vi "4Pi 4Pi Modes Control.vi"(7 "Calling VI Ref":refnum<vi>) -> ()   [LabVIEW 2016]
uses:
  4Pi 4Pi Modes - Controls/4Pi 4Pi Modes - Mirror Modes.ctl
  4Pi 4Pi Modes - Controls/4Pi 4Pi Modes - Standard Action.ctl
  <vilib>/Utility/miscctls.llb/LVPointTypeDef.ctl
  Hardware Configuration/Hardware Configuration Controls/Standard Action.ctl
  <vilib>/Analysis/baseanly.llb/Mean (DBL).vi
  <vilib>/Analysis/NI_AALBase.lvlib
  <userlib>/BMC/BMC.lvlib
panel:
  in  "Clear Flat":bool
  in  "Select Modes":bool
  in  "No Hardware":bool
  in  "Add Flat":bool
  out "?":string="Idel"
  out "?":string="Idel"
  in  "Set Astig":bool
  in  "Save Astig":bool
  out "Pixel Map (-1 to 1) 2":dbl[][](graph)
  in  "Scan Modes":bool
  in  "Astig On/Off":bool
  in  "Load Astig":bool
  in  "Clear Modes":bool
  in  "Mirror Modes":T1
  in  "Load Flat":bool
  in  "Save Flat":bool
  in  "Apply Flat":bool
  in  "Quit":bool
  out "Pixel Map (-1 to 1)":dbl[][](graph)
  # "Mode"
  # "Amount (nm)"
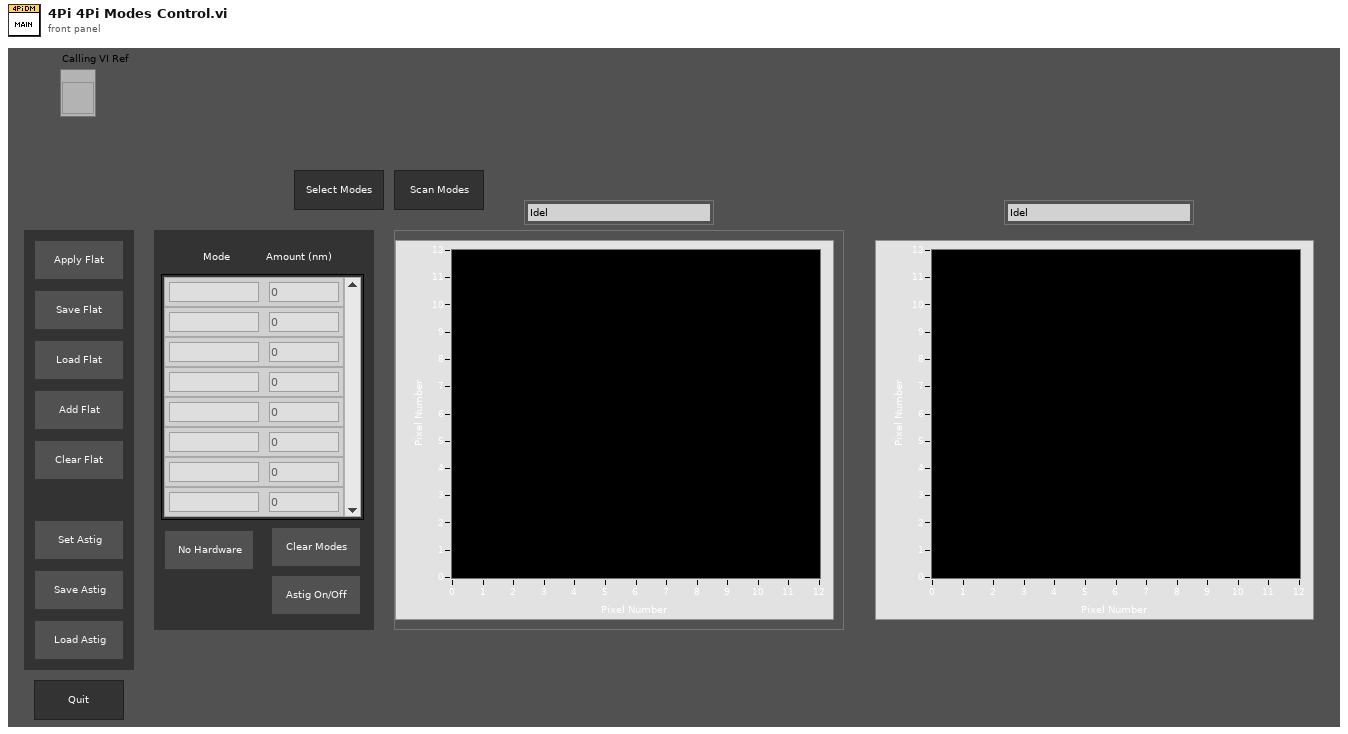
[diagram p1: front panel]
types:
  T1 = typedef "4Pi 4Pi Modes - Mirror Modes.ctl" = cluster{"Mode":string, "Amplitude":dbl}[]
  T2 = enum16{"Always On", "Always Off", "Off While Running"}
  T3 = typedef "LVPointTypeDef.ctl" = cluster{"Horizontal":i16, "Vertical":i16}
  T4 = typedef "4Pi 4Pi Modes - Standard Action.ctl" = enum16{"Read", "Write"}
  T5 = cluster{"type":i16, "ID":i16, "size":i32, "lutName":u64, "priv":u64}[]
  T6 = typedef "Standard Action.ctl" = enum16{"Read", "Write"}
  T7 = typedef "LVRectTypeDef.ctl" = cluster{"Left":i16, "Top":i16, "Right":i16, "Bottom":i16}
  T8 = typedef "LVBoundsTypeDef.ctl" = cluster{"Width":u32, "Height":u32}
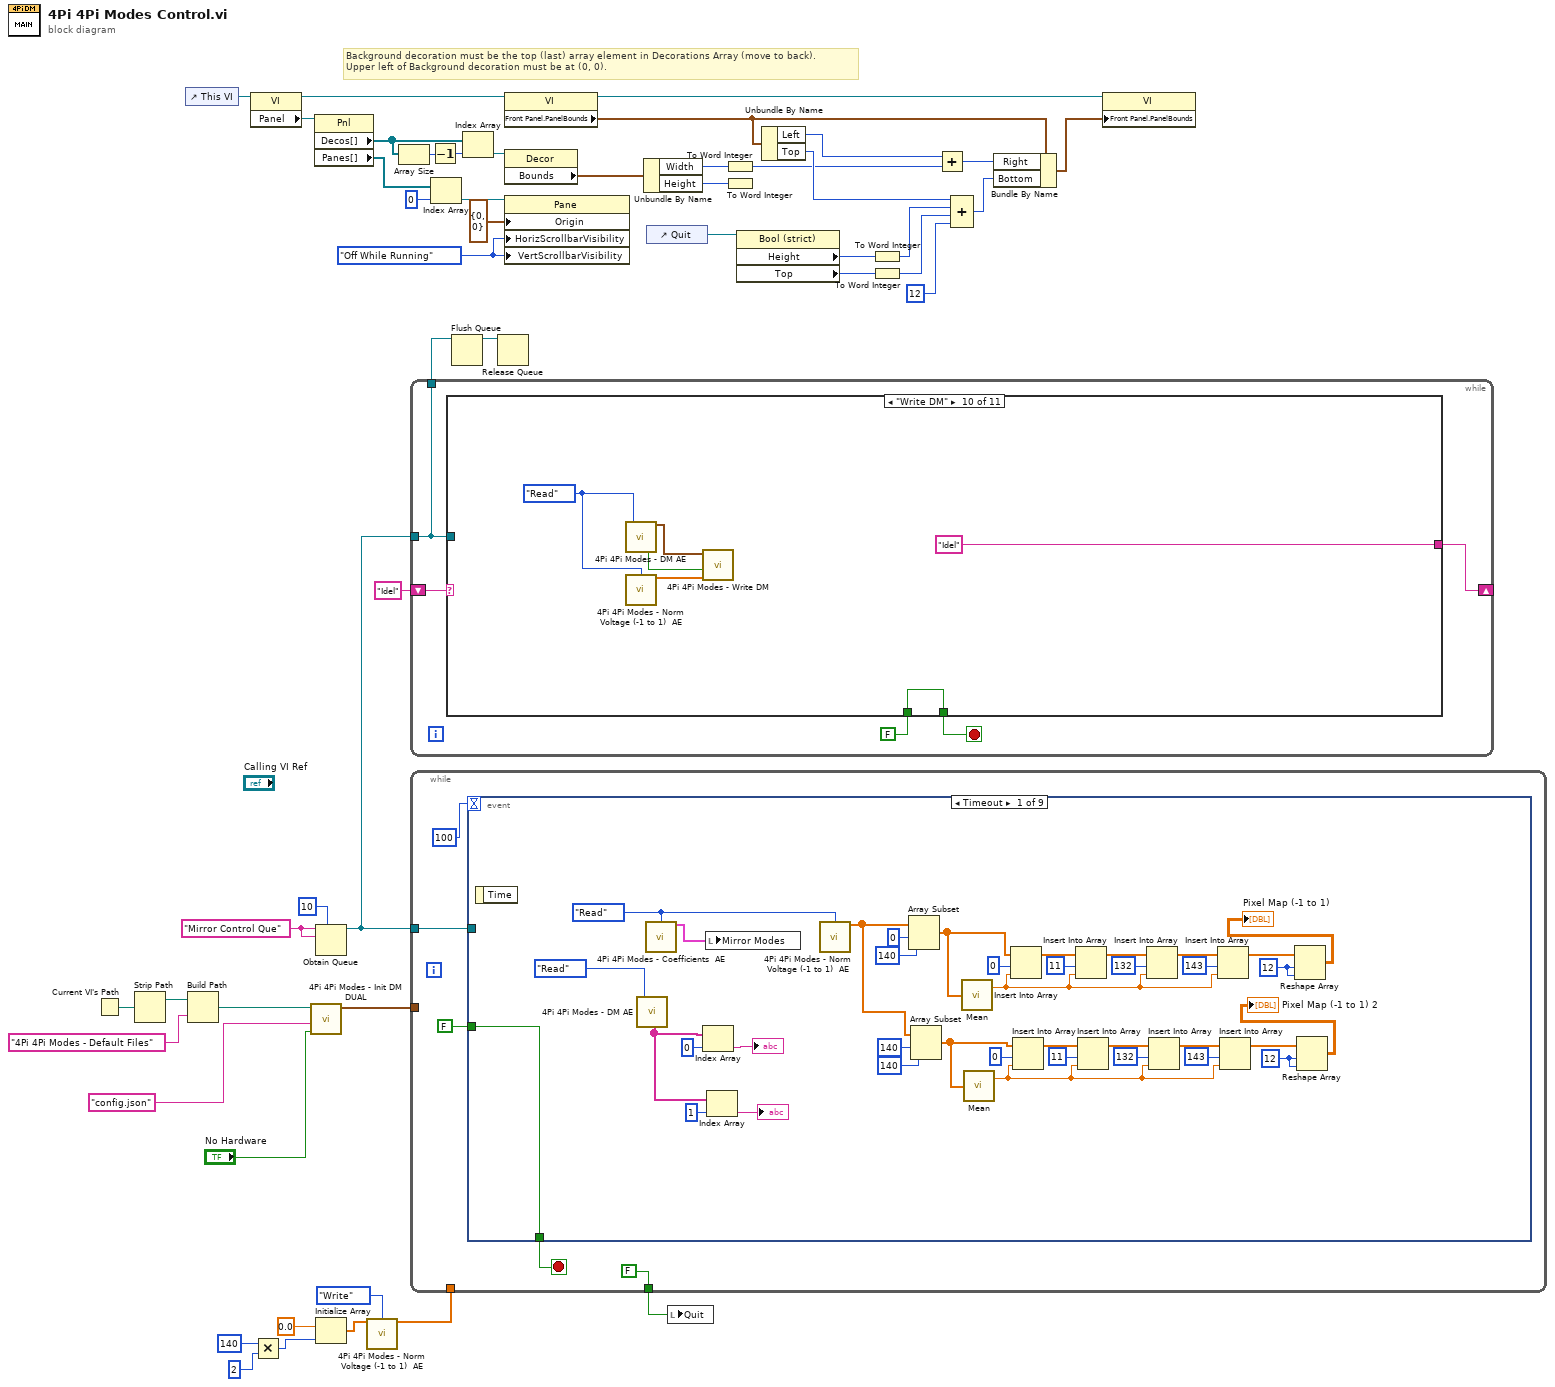
[diagram p0: block diagram]
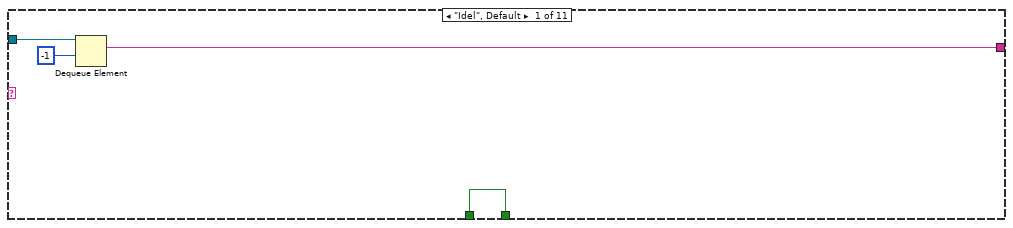
[diagram p2: hidden frame]
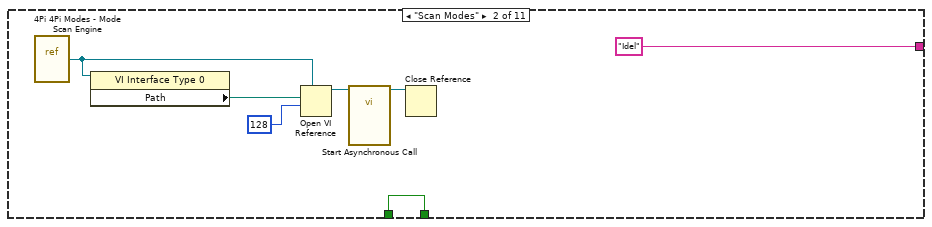
[diagram p3: hidden frame]
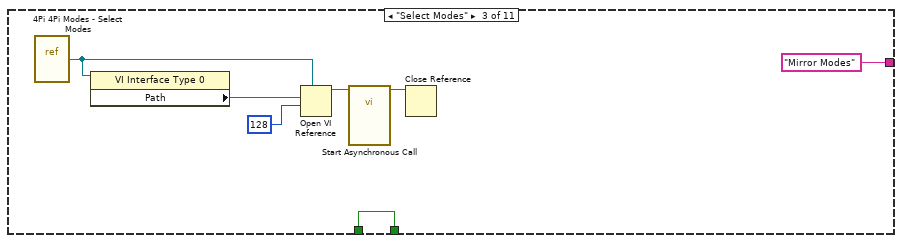
[diagram p4: hidden frame]
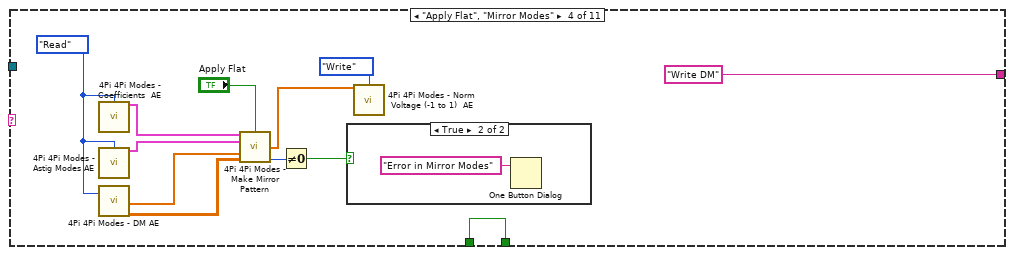
[diagram p5: hidden frame]
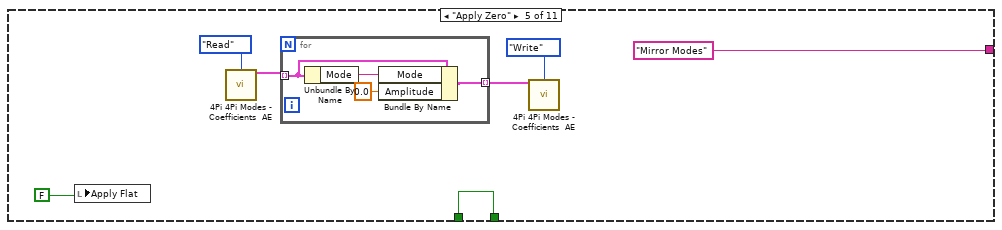
[diagram p7: hidden frame]
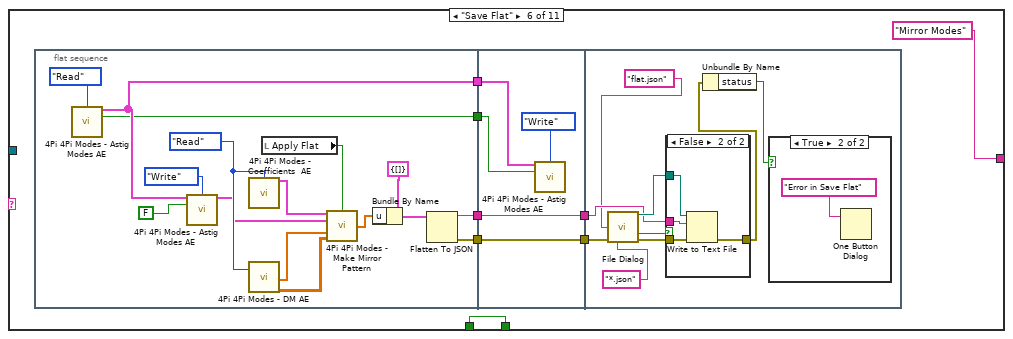
[diagram p8: hidden frame]
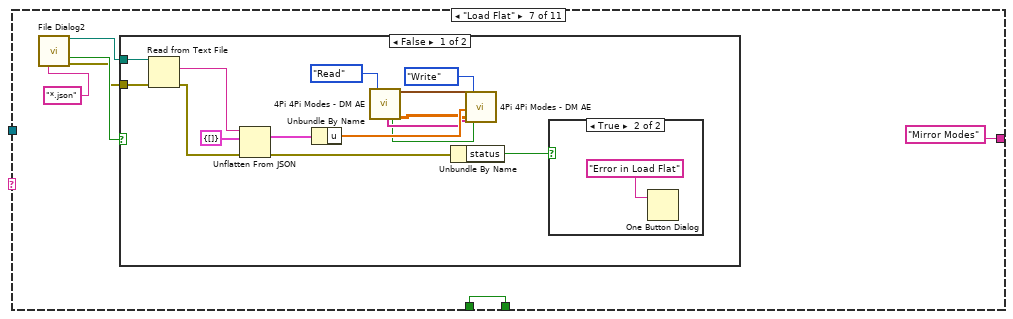
[diagram p11: hidden frame]
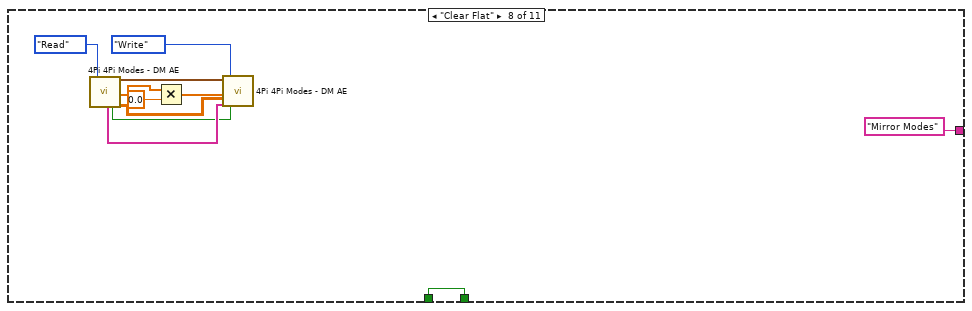
[diagram p14: hidden frame]
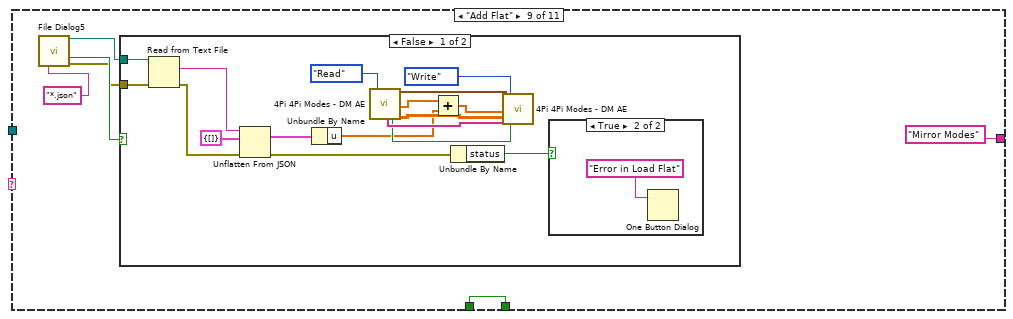
[diagram p15: hidden frame]
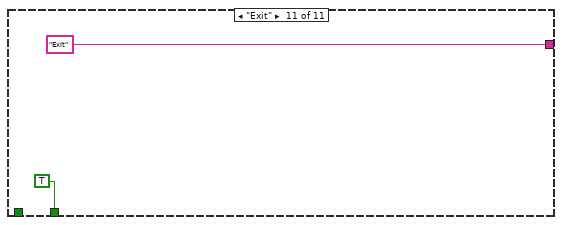
[diagram p18: hidden frame]
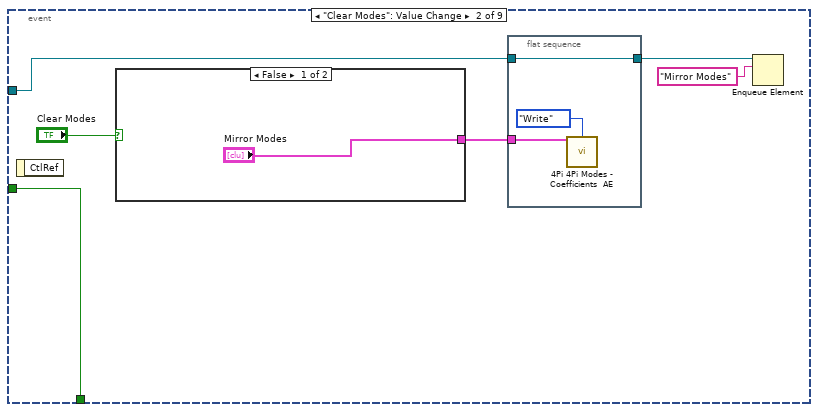
[diagram p19: hidden frame]
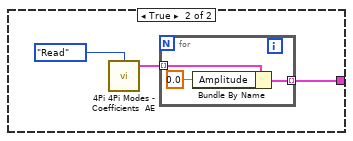
[diagram p20: hidden frame]
diagram:
  w24 = T2."Off While Running" ("Vertical Scrollbar Visibility")
  w50 = "Mirror Control Que" ("name (unnamed)")
  # "Background decoration must be the top (last) array element in Decorations Array (move to back).\nUpper left of Background decoration must be at (0, 0)."
  n1 = Current VI's Path() -> (path=w5:path)
  n2 = Strip Path(path=w5) -> (stripped path=w4:path)  [unwired: 1 out]
  n3 = control-ref of="This VI"() -> (w16:refnum<vi>)
  n4 = Build Path(base path=w4, name or relative path="4Pi 4Pi Modes - Default Files") -> (appended path=w2:path)
  n5 = property class="VI"(reference=w16) -> (reference out=w25:refnum<vi>, "Panel"=w17:refnum<vi>)  [unwired: 1 in, 1 out]
  n6 = Multiply(x=140 ("dimension size"), y=2 ("dimension size")) -> (x*y=w9:i32)
  n7 = call "4Pi 4Pi Modes - Init DM DUAL.vi"("No hardware"="No Hardware", "Config File"="config.json" ("name or relative path"), "Base File Path"=w2) -> ("DM Handles"=w48:T5)  [unwired: 7 in, 1 out]
  n8 = property class="Pnl"(reference=w17) -> ("Decos[]"=w15:refnum<vi>[], "Panes[]"=w21:refnum<vi>[])  [unwired: 1 in, 2 out]
  n9 = Obtain Queue(max queue size (-1, unlimited)=10, name (unnamed)=w50, element data type=w50) -> (queue out=w44:refnum<queue>)  [unwired: 2 in, 2 out]
  n10 = Initialize Array(0.0 ("element"), w9) -> (w8:dbl[])
  n11 = call "4Pi 4Pi Modes - Norm Voltage (-1 to 1)  AE.vi"("Pixel Value (-1 to 1)"=w8, "Action"=4Pi_4Pi_Modes_-_Standard_Action."Write") -> ("Pixel Value (-1 to 1) Out"=w7:dbl[])  [unwired: 13 in]
  n12 = Array Size(array=w15) -> (size(s)=w13:i32)
  n13 = while {
    tunnel: w44 -> [w51]
    shift-right: [w55] -> _
    shift-left: "Idel" ("name (unnamed)") -> [w54]
    tunnel: [w51] -> w47
    stop <- w53 stop-if-true
    n14 = case shown="\"Write DM\"" w54 {
      tunnel: w51 -> [w59 _ _ _ _ _ _ _ _ _ _]
      tunnel: [w57 "Idel" ("name (unnamed)") "Mirror Modes" ("name (unnamed)") "Write DM" ("name (unnamed)") "Mirror Modes" ("name (unnamed)") "Mirror Modes" ("name (unnamed)") "Mirror Modes" ("name (unnamed)") "Mirror Modes" ("name (unnamed)") "Mirror Modes" ("name (unnamed)") "Idel" ("name (unnamed)") "Exit" ("name (unnamed)")] -> w55
      tunnel: [w56 w66 w73 w84 w93 w105 w147 w174 w180 w204 TRUE] -> w53
      tunnel: FALSE -> [w56 w66 w73 w84 w93 w105 w147 w174 w180 w204 _]
      frame "Idel", Default {
        n15 = Dequeue Element(queue=w59, timeout in ms (-1)=-1) -> (element=w57:string)  [unwired: 1 in, 3 out]
      }
      frame "Scan Modes" {
        n16 = vi-ref "4Pi 4Pi Modes - Mode Scan Engine.vi"() -> (w60:refnum<vi>)
        n17 = property class="VI Interface Type 0"(reference=w60) -> ("Path"=w61:path)  [unwired: 1 in, 2 out]
        n18 = Open VI Reference(type specifier VI Refnum (for type only)=w60, vi path=w61, options=128) -> (vi reference=w63:refnum<vi>)  [unwired: 3 in, 1 out]
        n19 = call-by-ref "Start Asynchronous Call"(reference=w63) -> (reference out=w64:refnum<vi>)  [unwired: 17 in, 1 out]
        n20 = Close Reference(reference=w64) -> ()  [unwired: 1 in, 1 out]
      }
      frame "Select Modes" {
        n21 = vi-ref "4Pi 4Pi Modes - Select Modes.vi"() -> (w67:refnum<vi>)
        n22 = property class="VI Interface Type 0"(reference=w67) -> ("Path"=w68:path)  [unwired: 1 in, 2 out]
        n23 = Open VI Reference(type specifier VI Refnum (for type only)=w67, vi path=w68, options=128) -> (vi reference=w70:refnum<vi>)  [unwired: 3 in, 1 out]
        n24 = call-by-ref "Start Asynchronous Call"(reference=w70) -> (reference out=w71:refnum<vi>)  [unwired: 17 in, 1 out]
        n25 = Close Reference(reference=w71) -> ()  [unwired: 1 in, 1 out]
      }
      frame "Apply Flat", "Mirror Modes" {
        w77 = 4Pi_4Pi_Modes_-_Standard_Action."Read" ("Action")
        n26 = call "4Pi 4Pi Modes - Coefficients  AE.vi"("Action"=w77) -> ("Coefficients Out"=w79:cluster{"Mode":string, "Amplitude":dbl}[])  [unwired: 14 in]
        n27 = call "4Pi 4Pi Modes - Astig Modes AE.vi"("Action"=w77) -> ("Coefficients Out"=w76:cluster{"Mode":string, "Amplitude":dbl}[])  [unwired: 13 in, 1 out]
        n28 = call "4Pi 4Pi Modes - DM AE.vi"("Action"=w77) -> ("Flats Out"=w78:dbl[], "Control Matrix Out"=w82:dbl[][])  [unwired: 14 in, 3 out]
        n29 = call "4Pi 4Pi Modes - Make Mirror Pattern.vi"("Coefficients"=w79, "Flat On?"="Apply Flat", "Astig Coeffs"=w76, "Flats"=w78, "Control Matrix"=w82) -> ("Pixel Value U (-1 to 1)"=w80:dbl[], "error"=w75:i32)  [unwired: 9 in]
        n30 = Not Equal To 0?(x=w75) -> (x != 0?=w74:bool)
        n31 = case shown="True" w74 {
          frame False {
          }
          frame True {
            n32 = One Button Dialog(message="Error in Mirror Modes") -> ()  [unwired: 1 in, 1 out]
          }
        }
        n33 = call "4Pi 4Pi Modes - Norm Voltage (-1 to 1)  AE.vi"("Pixel Value (-1 to 1)"=w80, "Action"=4Pi_4Pi_Modes_-_Standard_Action."Write") -> ()  [unwired: 13 in, 1 out]
      }
      frame "Apply Zero" {
        n34 = local write "Apply Flat"(FALSE ("Apply Flat")) -> ()
        n35 = call "4Pi 4Pi Modes - Coefficients  AE.vi"("Action"=4Pi_4Pi_Modes_-_Standard_Action."Read") -> ("Coefficients Out"=w89:cluster{"Mode":string, "Amplitude":dbl}[])  [unwired: 14 in]
        n36 = for {
          tunnel: w89 -> [w96] mode=indexing
          tunnel: [w94] -> w87 mode=indexing
          n37 = Unbundle By Name(w96) -> ("Mode"=w97:string)
          n38 = Bundle By Name(cluster=w96, "Mode"=w97, "Amplitude"=0.0) -> (w94:cluster{"Mode":string, "Amplitude":dbl})
        }
        n39 = call "4Pi 4Pi Modes - Coefficients  AE.vi"("Coefficients In"=w87, "Action"=4Pi_4Pi_Modes_-_Standard_Action."Write") -> ()  [unwired: 13 in, 1 out]
      }
      frame "Save Flat" {
        n40 = flat-sequence {
          tunnel: [w109] -> w103
          tunnel: [w108] -> w102
          tunnel: [w107] -> w100
          tunnel: [w106] -> w98
          tunnel: w103 -> [w125]
          tunnel: w102 -> [w124]
          tunnel: [w123] -> w101
          tunnel: w100 -> [w123]
          tunnel: [w122] -> w99
          tunnel: w98 -> [w122]
          tunnel: w101 -> [w135]
          tunnel: w99 -> [w131]
          frame #0 {
            w118 = 4Pi_4Pi_Modes_-_Standard_Action."Read" ("Action")
            n41 = call "4Pi 4Pi Modes - Astig Modes AE.vi"("Action"=Standard_Action."Read") -> ("Coefficients Out"=w109:cluster{"Mode":string, "Amplitude":dbl}[], "Enabled Out"=w108:bool)  [unwired: 13 in]
            n42 = call "4Pi 4Pi Modes - Astig Modes AE.vi"("Coefficients In"=w109, "Action"=Standard_Action."Write", "Enabled In"=FALSE) -> ("Coefficients Out"=w116:cluster{"Mode":string, "Amplitude":dbl}[])  [unwired: 11 in, 1 out]
            n43 = call "4Pi 4Pi Modes - Coefficients  AE.vi"("Action"=w118) -> ("Coefficients Out"=w117:cluster{"Mode":string, "Amplitude":dbl}[])  [unwired: 14 in]
            n44 = call "4Pi 4Pi Modes - DM AE.vi"("Action"=w118) -> ("Flats Out"=w115:dbl[], "Control Matrix Out"=w114:dbl[][])  [unwired: 14 in, 3 out]
            n45 = local read "Apply Flat"() -> (w113:bool)
            n46 = call "4Pi 4Pi Modes - Make Mirror Pattern.vi"("Coefficients"=w117, "Flat On?"=w113, "Astig Coeffs"=w116, "Flats"=w115, "Control Matrix"=w114) -> ("Pixel Value U (-1 to 1)"=w111:dbl[])  [unwired: 9 in, 1 out]
            n47 = Bundle By Name(cluster=cluster{"u":dbl[]} {"u"=[]}, "u"=w111) -> (w110:cluster{"u":dbl[]})
            n48 = Flatten To JSON(anything=w110) -> (JSON string=w106:string, 11:w107:errorcluster)  [unwired: 2 in]
          }
          frame #1 {
            n49 = call "4Pi 4Pi Modes - Astig Modes AE.vi"("Coefficients In"=w125, "Action"=Standard_Action."Write", "Enabled In"=w124) -> ()  [unwired: 11 in, 2 out]
          }
          frame #2 {
            n50 = call "File Dialog"("default name"="flat.json", "error in"=w135, "pattern (all files)"="*.json") -> ("selected path"=w132:path, "cancelled"=w133:bool, "error out"=w134:errorcluster)  [unwired: 9 in, 1 out]
            n51 = case shown="False" w133 {
              tunnel: w134 -> [w137 w141]
              tunnel: w132 -> [_ w140]
              tunnel: w131 -> [_ w139]
              tunnel: [w137 w138] -> w130
              frame True {
              }
              frame False {
                n52 = Write to Text File(file (use dialog)=w140, text=w139, error in=w141) -> (error out=w138:errorcluster)  [unwired: 1 in, 2 out]
              }
            }
            n53 = Unbundle By Name(w130) -> ("status"=w129:bool)
            n54 = case shown="True" w129 {
              frame False {
              }
              frame True {
                n55 = One Button Dialog(message="Error in Save Flat") -> ()  [unwired: 1 in, 1 out]
              }
            }
          }
        }
      }
      frame "Load Flat" {
        n56 = call "File Dialog2"("pattern (all files)"="*.json") -> ("selected path"=w143:path, "cancelled"=w145:bool, "error out"=w144:errorcluster)  [unwired: 11 in, 1 out]
        n57 = case shown="False" w145 {
          tunnel: w144 -> [w162 _]
          tunnel: w143 -> [w161 _]
          frame False {
            n58 = Read from Text File(file (use dialog)=w161, error in=w162) -> (text=w160:string, error out=w159:errorcluster)  [unwired: 2 in, 2 out]
            n59 = Unflatten From JSON(JSON string=w160, type and defaults=cluster{"u":dbl[]} {"u"=[]}, error in (no error)=w159) -> (value=w157:cluster{"u":dbl[]}, error out=w150:errorcluster)  [unwired: 4 in]
            n60 = Unbundle By Name(w157) -> ("u"=w153:dbl[])
            n61 = call "4Pi 4Pi Modes - DM AE.vi"("Action"=4Pi_4Pi_Modes_-_Standard_Action."Read") -> ("Serials Out"=w149:string[], "No hardware Out"=w148:bool, "DM Handles Out"=w154:T5, "Control Matrix Out"=w152:dbl[][])  [unwired: 14 in, 1 out]
            n62 = Unbundle By Name(w150) -> ("status"=w151:bool)
            n63 = call "4Pi 4Pi Modes - DM AE.vi"("DM Handles"=w154, "Flats"=w153, "Control Matrix"=w152, "Serials"=w149, "Action"=4Pi_4Pi_Modes_-_Standard_Action."Write", "No hardware"=w148) -> ()  [unwired: 9 in, 5 out]
            n64 = case shown="True" w151 {
              frame False {
              }
              frame True {
                n65 = One Button Dialog(message="Error in Load Flat") -> ()  [unwired: 1 in, 1 out]
              }
            }
          }
          frame True {
          }
        }
      }
      frame "Clear Flat" {
        n66 = call "4Pi 4Pi Modes - DM AE.vi"("Action"=4Pi_4Pi_Modes_-_Standard_Action."Read") -> ("Serials Out"=w165:string[], "No hardware Out"=w164:bool, "DM Handles Out"=w170:T5, "Flats Out"=w168:dbl[], "Control Matrix Out"=w166:dbl[][])  [unwired: 14 in]
        n67 = Multiply(x=w168, y=0.0) -> (x*y=w167:dbl[])
        n68 = call "4Pi 4Pi Modes - DM AE.vi"("DM Handles"=w170, "Flats"=w167, "Control Matrix"=w166, "Serials"=w165, "Action"=4Pi_4Pi_Modes_-_Standard_Action."Write", "No hardware"=w164) -> ()  [unwired: 9 in, 5 out]
      }
      frame "Add Flat" {
        n69 = call "File Dialog5"("pattern (all files)"="*.json") -> ("selected path"=w176:path, "cancelled"=w178:bool, "error out"=w177:errorcluster)  [unwired: 11 in, 1 out]
        n70 = case shown="False" w178 {
          tunnel: w177 -> [w197 _]
          tunnel: w176 -> [w196 _]
          frame False {
            n71 = Read from Text File(file (use dialog)=w196, error in=w197) -> (text=w195:string, error out=w194:errorcluster)  [unwired: 2 in, 2 out]
            n72 = Unflatten From JSON(JSON string=w195, type and defaults=cluster{"u":dbl[]} {"u"=[]}, error in (no error)=w194) -> (value=w192:cluster{"u":dbl[]}, error out=w186:errorcluster)  [unwired: 4 in]
            n73 = Unbundle By Name(w192) -> ("u"=w181:dbl[])
            n74 = call "4Pi 4Pi Modes - DM AE.vi"("Action"=4Pi_4Pi_Modes_-_Standard_Action."Read") -> ("Serials Out"=w185:string[], "No hardware Out"=w184:bool, "DM Handles Out"=w189:T5, "Flats Out"=w182:dbl[], "Control Matrix Out"=w188:dbl[][])  [unwired: 14 in]
            n75 = Add(x=w182, y=w181) -> (x+y=w183:dbl[])
            n76 = Unbundle By Name(w186) -> ("status"=w187:bool)
            n77 = call "4Pi 4Pi Modes - DM AE.vi"("DM Handles"=w189, "Flats"=w183, "Control Matrix"=w188, "Serials"=w185, "Action"=4Pi_4Pi_Modes_-_Standard_Action."Write", "No hardware"=w184) -> ()  [unwired: 9 in, 5 out]
            n78 = case shown="True" w187 {
              frame False {
              }
              frame True {
                n79 = One Button Dialog(message="Error in Load Flat") -> ()  [unwired: 1 in, 1 out]
              }
            }
          }
          frame True {
          }
        }
      }
      frame "Write DM" {
        w202 = 4Pi_4Pi_Modes_-_Standard_Action."Read" ("Action")
        n80 = call "4Pi 4Pi Modes - DM AE.vi"("Action"=w202) -> ("No hardware Out"=w199:bool, "DM Handles Out"=w201:T5)  [unwired: 14 in, 3 out]
        n81 = call "4Pi 4Pi Modes - Norm Voltage (-1 to 1)  AE.vi"("Action"=w202) -> ("Pixel Value (-1 to 1) Out"=w200:dbl[])  [unwired: 14 in]
        n82 = call "4Pi 4Pi Modes - Write DM.vi"("DM Handles"=w201, "No hardware"=w199, "Norm Voltage (-1, 1)"=w200) -> ()  [unwired: 4 in, 1 out]
      }
      frame "Exit" {
      }
    }
  }
  n83 = while {
    tunnel: w44 -> [w208]
    tunnel: w48 -> [_]
    tunnel: [FALSE] -> w12
    tunnel: w7 -> [_]
    stop <- w211 stop-if-true
    n84 = event shown="[0] Timeout" {
      selector: _ -> [_ _ _ _ _ _ _ _ _]
      dyn-events: _ -> [_ _ _ _ _ _ _ _ _]
      timeout: 100 -> [_ _ _ _ _ _ _ _ _]
      tunnel: [w249 w255 w271 w278 w284 _ _ w333 w347] -> w211
      tunnel: FALSE -> [w249 w255 w271 w278 w284 _ _ w333 _]
      tunnel: w208 -> [_ w254 w270 w277 w280 _ w324 w332 w346]
      event Timeout {
        w236 = 12 ("dimension size")
        w247 = 12 ("dimension size")
        w248 = 4Pi_4Pi_Modes_-_Standard_Action."Read" ("Action")
        n85 = event-data() -> ()  [unwired: 1 in, 1 out]
        n86 = call "4Pi 4Pi Modes - DM AE.vi"("Action"=4Pi_4Pi_Modes_-_Standard_Action."Read") -> ("Serials Out"=w214:string[])  [unwired: 14 in, 4 out]
        n87 = call "4Pi 4Pi Modes - Coefficients  AE.vi"("Action"=w248) -> ("Coefficients Out"=w225:cluster{"Mode":string, "Amplitude":dbl}[])  [unwired: 14 in]
        n88 = Index Array(array=w214, index=0) -> (element=→"?":string)
        n89 = local write "Mirror Modes"(w225) -> ()
        n90 = Index Array(array=w214, index=1) -> (element=→"?":string)
        n91 = call "4Pi 4Pi Modes - Norm Voltage (-1 to 1)  AE.vi"("Action"=w248) -> ("Pixel Value (-1 to 1) Out"=w220:dbl[])  [unwired: 14 in]
        n92 = Array Subset(array=w220, index=0, length=140) -> (w218:dbl[])
        n93 = Array Subset(array=w220, index=140, length=140) -> (w219:dbl[])
        n94 = call-poly <vilib>:"Mean.vi"("X"=w218) -> ("mean"=w245:dbl)  [unwired: 1 out]
        n95 = call-poly <vilib>:"Mean.vi"("X"=w219) -> ("mean"=w235:dbl)  [unwired: 1 out]
        n96 = Insert Into Array(array=w218, index=0, new element=w245) -> (w240:dbl[])
        n97 = Insert Into Array(array=w219, index=0, new element=w235) -> (w230:dbl[])
        n98 = Insert Into Array(array=w240, index=11, new element=w245) -> (w242:dbl[])
        n99 = Insert Into Array(array=w230, index=11, new element=w235) -> (w232:dbl[])
        n100 = Insert Into Array(array=w242, index=132, new element=w245) -> (w244:dbl[])
        n101 = Insert Into Array(array=w232, index=132, new element=w235) -> (w234:dbl[])
        n102 = Insert Into Array(array=w244, index=143, new element=w245) -> (w237:dbl[])
        n103 = Insert Into Array(array=w234, index=143, new element=w235) -> (w227:dbl[])
        n104 = Reshape Array(w237, w247, w247) -> (→"Pixel Map (-1 to 1)":dbl[][])
        n105 = Reshape Array(w227, w236, w236) -> (→"Pixel Map (-1 to 1) 2":dbl[][])
      }
      event "Clear Modes": Value Change {
        n106 = event-data() -> ()  [unwired: 1 in, 1 out]
        n107 = case shown="False" "Clear Modes" {
          tunnel: ["Mirror Modes" w257] -> w250
          frame False {
          }
          frame True {
            n108 = call "4Pi 4Pi Modes - Coefficients  AE.vi"("Action"=4Pi_4Pi_Modes_-_Standard_Action."Read") -> ("Coefficients Out"=w258:cluster{"Mode":string, "Amplitude":dbl}[])  [unwired: 14 in]
            n109 = for {
              tunnel: [w261] -> w257 mode=indexing
              tunnel: w258 -> [w260] mode=indexing
              n110 = Bundle By Name(cluster=w260, "Amplitude"=0.0) -> (w261:cluster{"Mode":string, "Amplitude":dbl})
            }
          }
        }
        n111 = flat-sequence {
          tunnel: w250 -> [w263]
          tunnel: w254 -> [w265]
          tunnel: [w265] -> w252
          frame #0 {
            n112 = call "4Pi 4Pi Modes - Coefficients  AE.vi"("Coefficients In"=w263, "Action"=4Pi_4Pi_Modes_-_Standard_Action."Write") -> ()  [unwired: 13 in, 1 out]
          }
        }
        n113 = Enqueue Element(queue=w252, element="Mirror Modes") -> ()  [unwired: 2 in, 3 out]
      }
      event "Add Flat", "Save Flat", "Load Flat", "Scan Modes", "Select Modes", "Clear Flat": Value Change {
        n114 = event-data() -> ("CtlRef"=w269:refnum<vi>, "OldVal"=w267:bool, "NewVal"=w268:bool)  [unwired: 1 in]
        n115 = Greater Or Equal?(x=w268, y=w267) -> (x >= y?=w266:bool)
        n116 = case shown="True" w266 {
          tunnel: w270 -> [_ w274]
          tunnel: w269 -> [_ w273]
          frame False {
          }
          frame True {
            n117 = property class="Bool"(reference=w273) -> ("Label.Text"=w272:string)  [unwired: 1 in, 2 out]
            n118 = Enqueue Element(queue=w274, element=w272) -> ()  [unwired: 2 in, 3 out]
          }
        }
      }
      event "Apply Flat": Value Change {
        n119 = event-data() -> ("CtlRef"=w276:refnum<vi>)  [unwired: 1 in]
        n120 = property class="Bool (strict)"(reference=w276) -> ("Label.Text"=w275:string)  [unwired: 1 in, 2 out]
        n121 = Enqueue Element(queue=w277, element=w275) -> ()  [unwired: 2 in, 3 out]
      }
      event "Load Astig": Value Change {
        n122 = event-data() -> ()  [unwired: 1 in, 1 out]
        n123 = call "File Dialog3"("pattern (all files)"="*.json") -> ("selected path"=w281:path, "cancelled"=w283:bool, "error out"=w282:errorcluster)  [unwired: 11 in, 1 out]
        n124 = case shown="False" w283 {
          tunnel: w282 -> [w287 _]
          tunnel: w281 -> [w286 _]
          tunnel: w280 -> [w285 _]
          frame False {
            n125 = flat-sequence {
              tunnel: w287 -> [w302]
              tunnel: w286 -> [w301]
              tunnel: w285 -> [w308]
              frame #0 {
                n126 = call "4Pi 4Pi Modes - Astig Modes AE.vi"("Action"=4Pi_4Pi_Modes_-_Standard_Action."Read") -> ("Coefficients Out"=w290:cluster{"Mode":string, "Amplitude":dbl}[], "Enabled Out"=w288:bool)  [unwired: 13 in]
                n127 = Read from Text File(file (use dialog)=w301, error in=w302) -> (text=w300:string, error out=w299:errorcluster)  [unwired: 2 in, 2 out]
                n128 = call "4Pi 4Pi Modes - Vectorise Coefficients.vi"("Coefficients In"=w290) -> ("Coefficients Out"=w289:cluster{"Amplitudes":dbl[], "Modes":string[]})  [unwired: 14 in]
                n129 = Unflatten From JSON(JSON string=w300, type and defaults=w289, error in (no error)=w299) -> (value=w294:cluster{"Amplitudes":dbl[], "Modes":string[]}, error out=w297:errorcluster)  [unwired: 4 in]
                n130 = Unbundle By Name(w294) -> ("Modes"=w293:string[], "Amplitudes"=w292:dbl[])
                n131 = Unbundle By Name(w297) -> ("status"=w298:bool)
                n132 = for {
                  tunnel: w290 -> [w306] mode=indexing
                  tunnel: w293 -> [w304] mode=indexing
                  tunnel: w292 -> [w303] mode=indexing
                  tunnel: [w305] -> w291 mode=indexing
                  n133 = Bundle By Name(cluster=w306, "Mode"=w304, "Amplitude"=w303) -> (w305:cluster{"Mode":string, "Amplitude":dbl})
                }
                n134 = case shown="True" w298 {
                  frame False {
                  }
                  frame True {
                    n135 = One Button Dialog(message="Error in Load Astig") -> ()  [unwired: 1 in, 1 out]
                  }
                }
                n136 = call "4Pi 4Pi Modes - Astig Modes AE.vi"("Coefficients In"=w291, "Action"=4Pi_4Pi_Modes_-_Standard_Action."Write", "Enabled In"=w288) -> ()  [unwired: 11 in, 2 out]
              }
              frame #1 {
                n137 = Enqueue Element(queue=w308, element="Mirror Modes") -> ()  [unwired: 2 in, 3 out]
              }
            }
          }
          frame True {
          }
        }
      }
      event "Save Astig": Value Change {
        n138 = event-data() -> ()  [unwired: 1 in, 1 out]
        n139 = call "File Dialog4"("pattern (all files)"="*.json") -> ("selected path"=w310:path, "cancelled"=w312:bool, "error out"=w311:errorcluster)  [unwired: 11 in, 1 out]
        n140 = case shown="False" w312 {
          tunnel: w311 -> [w319 _]
          tunnel: w310 -> [w317 _]
          frame False {
            n141 = call "4Pi 4Pi Modes - Astig Modes AE.vi"("Action"=4Pi_4Pi_Modes_-_Standard_Action."Read") -> ("Coefficients Out"=w321:cluster{"Mode":string, "Amplitude":dbl}[])  [unwired: 13 in, 1 out]
            n142 = call "4Pi 4Pi Modes - Vectorise Coefficients.vi"("Coefficients In"=w321) -> ("Coefficients Out"=w320:cluster{"Amplitudes":dbl[], "Modes":string[]})  [unwired: 14 in]
            n143 = Flatten To JSON(anything=w320, error in (no error)=w319) -> (JSON string=w318:string, 11:w316:errorcluster)  [unwired: 1 in]
            n144 = Write to Text File(file (use dialog)=w317, text=w318, error in=w316) -> (error out=w314:errorcluster)  [unwired: 1 in, 2 out]
            n145 = Unbundle By Name(w314) -> ("status"=w315:bool)
            n146 = case shown="True" w315 {
              frame False {
              }
              frame True {
                n147 = One Button Dialog(message="Error in Save Astig") -> ()  [unwired: 1 in, 1 out]
              }
            }
          }
          frame True {
          }
        }
      }
      event "Set Astig": Value Change {
        # "Store the current DM state into the astigmatism AE"
        n148 = event-data() -> ()  [unwired: 1 in, 1 out]
        n149 = flat-sequence {
          tunnel: w324 -> [w330]
          frame #0 {
            n150 = call "4Pi 4Pi Modes - Coefficients  AE.vi"("Action"=4Pi_4Pi_Modes_-_Standard_Action."Read") -> ("Coefficients Out"=w327:cluster{"Mode":string, "Amplitude":dbl}[])  [unwired: 14 in]
            n151 = call "4Pi 4Pi Modes - Astig Modes AE.vi"("Action"=Standard_Action."Read") -> ("Enabled Out"=w325:bool)  [unwired: 13 in, 1 out]
            n152 = call "4Pi 4Pi Modes - Astig Modes AE.vi"("Coefficients In"=w327, "Action"=Standard_Action."Write", "Enabled In"=w325) -> ()  [unwired: 11 in, 2 out]
          }
          frame #1 {
            n153 = Enqueue Element(queue=w330, element="Mirror Modes") -> ()  [unwired: 2 in, 3 out]
          }
        }
      }
      event "Astig On/Off": Value Change {
        n154 = event-data() -> ()  [unwired: 1 in, 1 out]
        n155 = flat-sequence {
          tunnel: w332 -> [w338]
          frame #0 {
            n156 = call "4Pi 4Pi Modes - Astig Modes AE.vi"("Action"=Standard_Action."Read") -> ("Coefficients Out"=w335:cluster{"Mode":string, "Amplitude":dbl}[])  [unwired: 13 in, 1 out]
            n157 = call "4Pi 4Pi Modes - Astig Modes AE.vi"("Coefficients In"=w335, "Action"=Standard_Action."Write", "Enabled In"="Astig On/Off") -> ()  [unwired: 11 in, 2 out]
          }
          frame #1 {
            n158 = Enqueue Element(queue=w338, element="Mirror Modes") -> ()  [unwired: 2 in, 3 out]
          }
        }
      }
      event "Quit": Value Change {
        n159 = event-data() -> ("NewVal"=w347:bool)  [unwired: 1 in]
        n160 = flat-sequence {
          tunnel: w346 -> [w360]
          tunnel: [w357] -> w343
          tunnel: [w356] -> w341
          frame #0 {
            n161 = call "4Pi 4Pi Modes - Norm Voltage (-1 to 1)  AE.vi"("Action"=4Pi_4Pi_Modes_-_Standard_Action."Read") -> ("Pixel Value (-1 to 1) Out"=w353:dbl[])  [unwired: 14 in]
            n162 = Multiply(x=w353, y=0.0 ("x*y")) -> (x*y=w352:dbl[])
            n163 = Add(x=w352, y=-1.0 ("x*y")) -> ()  [unwired: 1 out]
          }
          frame #1 {
            n164 = Wait (ms)(milliseconds to wait=u32 300) -> ()  [unwired: 1 out]
            n165 = Enqueue Element(queue=w360, element="Write DM") -> (queue out=w357:refnum<queue>, error out=w356:errorcluster)  [unwired: 2 in, 1 out]
          }
        }
        n166 = Enqueue Element(queue=w343, element="Exit", error in (no error)=w341) -> (error out=w340:errorcluster)  [unwired: 1 in, 2 out]
        n167 = call "4Pi 4Pi Modes - DM AE.vi"("Action"=4Pi_4Pi_Modes_-_Standard_Action."Read") -> ("DM Handles Out"=w342:T5)  [unwired: 14 in, 4 out]
        n168 = for {
          tunnel: w342 -> [w350] mode=indexing
          tunnel: [w349] -> _ mode=indexing
          tunnel: w340 -> [w348]
          n169 = call <userlib>:"BMC Close DM.vi"("error in (no error)"=w348, "dmHandle"=w350) -> ("function return"=w349:i32)  [unwired: 8 in, 1 out]
        }
      }
    }
  }
  n170 = Decrement(x=w13) -> (x-1=w14:i32)
  n171 = Index Array(array=w21, index=0) -> (element=w20:refnum<vi>)
  n172 = Flush Queue(queue=w47) -> (queue out=w46:refnum<queue>)  [unwired: 1 in, 2 out]
  n173 = Index Array(array=w15, index=w14) -> (element=w23:refnum<vi>)
  n174 = Release Queue(queue=w46) -> ()  [unwired: 2 in, 3 out]
  n175 = property class="VI"(reference=w25) -> (reference out=w27:refnum<vi>, "Front Panel.PanelBounds"=w28:T7)  [unwired: 1 in, 1 out]
  n176 = property class="Decor"(reference=w23) -> ("Bounds"=w26:T8)  [unwired: 1 in, 2 out]
  n177 = property class="Pane"(reference=w20, "Origin"=T3 {"Horizontal"=0, "Vertical"=0}, "HorizScrollbarVisibility"=w24, "VertScrollbarVisibility"=w24) -> ()  [unwired: 1 in, 2 out]
  n178 = Unbundle By Name(w26) -> ("Width"=w31:u32, "Height"=w34:u32)
  n179 = control-ref of="Quit"() -> (w18:refnum<vi>)
  n180 = local write "Quit"(w12) -> ()
  n181 = To Word Integer(number=w31) -> (16bit integer=w33:i16)
  n182 = To Word Integer(number=w34) -> ()  [unwired: 1 out]
  n183 = property class="Bool (strict)"(reference=w18) -> ("Height"=w36:u32, "Top"=w37:i32)  [unwired: 1 in, 2 out]
  n184 = Unbundle By Name(w28) -> ("Left"=w30:i16, "Top"=w41:i16)
  n185 = To Word Integer(number=w36) -> (16bit integer=w39:i16)
  n186 = To Word Integer(number=w37) -> (16bit integer=w40:i16)
  n187 = Add(x=w30, y=w33) -> (x+y=w32:i16)
  n188 = Compound Arithmetic op=ADD(w41, w39, w40, i16 12 ("y")) -> (w35:i16)
  n189 = Bundle By Name(cluster=w28, "Right"=w32, "Bottom"=w35) -> (w29:T7)
  n190 = property class="VI"(reference=w27, "Front Panel.PanelBounds"=w29) -> ()  [unwired: 1 in, 2 out]
